vi "Enable-Disable MovCor UI.vi"(10 "MC Supported":bool) -> ()   [LabVIEW 2020]
uses:
  Global Variables/gl_UI Ctrl Refs.vi
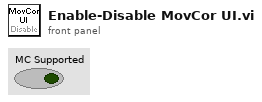
[diagram p1: front panel]
types:
  T1 = typedef "UI ctrl refs cluster.ctl" = cluster{"Top level VI path":path, "Top level VI ref":refnum<vi>, "User menu ref":refnum<k9>, "Sub Panel control":refnum<vi>, "Imaging Param Tab":refnum<vi>, "Occurrence-Start drivers":refnum<k4>, "Occurrence-Speed logging initialised":refnum<k4>, "Occurrence-XYZ stage initialised":refnum<k4>, "Exit button":refnum<vi>, "Status ind":refnum<vi>, "Set as origin":refnum<vi>, "Speed Logging":refnum<vi>, "Time Lapse":refnum<vi>, "Live Imaging":refnum<vi>, "AOL Z Stack":refnum<vi>, "Motor Z Stack":refnum<vi>, "Funct Acq button":refnum<vi>, "Hard Shutter":refnum<vi>, "Virtual Shutter":refnum<vi>, "Laser Power":refnum<vi>, "AOL Mode":refnum<vi>, "Frame Size":refnum<vi>, "Field of View":refnum<vi>, "Dwell Time":refnum<vi>, "Zoom":refnum<vi>, "AOL Z":refnum<vi>, "Objective":refnum<vi>, "Axis":refnum<vi>, "Paths & Names":refnum<vi>, "Experiment folder path (ind.)":refnum<vi>, "Last State (Ind.)":refnum<vi>, "Averages":refnum<vi>, "Angle (degrees)":refnum<vi>, "X centre":refnum<vi>, "Y centre":refnum<vi>, "Plane Mode":refnum<vi>, "# Planes":refnum<vi>, "Z Start":refnum<vi>, "Z Stop":refnum<vi>, "Z Step":refnum<vi>, "PMT 1":refnum<vi>, "PMT 2":refnum<vi>, "Stage XYZ Position":refnum<vi>, "Pockels@Z Start":refnum<vi>, "Pockels@Z Stop":refnum<vi>, "Obtain Z Start":refnum<vi>, "Obtain Z Stop":refnum<vi>, "Live stim.trig.period":refnum<vi>, "Live stim.trig.enable":refnum<vi>, "Movement Correction":refnum<vi>, "Load Reference Image":refnum<vi>, "XY Stage Move":refnum<vi>, "MovCor Cluster":refnum<vi>, "RefDAQParam":refnum<vi>, "Funct. Acq. Pockels Modulation":refnum<vi>, "Ref Laser Power":refnum<vi>, "Enable Video Recording":refnum<vi>, "Video Record-Live Imaging":refnum<vi>, "Video Record-Funct acq":refnum<vi>, "Reference Source":refnum<vi>, "AOL Z-stack Chirps Ready (ind)":refnum<vi>, "Target time between mov.cor. ref triggers (ms)":refnum<vi>, "Funct. Acq. Ref frame save":refnum<vi>, "Tracking button":refnum<vi>, "Show ref plots window":refnum<vi>, "Center freq ind (nm)":refnum<vi>, "Pickup mode (ind)":refnum<vi>, "Logging queue (ind)":refnum<vi>, "Back aperture power (ind.)":refnum<vi>, "Power after objective (ind.)":refnum<vi>, "Switch user":refnum<vi>, "Ls1 Conn. Status":refnum<vi>, "Ls1Tuning Status":refnum<vi>, "Ls1 Faults":refnum<vi>, "Ls1 Connection":refnum<vi>, "Ls1 Mode":refnum<vi>, "Ls1 POWER [mW]":refnum<vi>, "Ls1Shutter":refnum<vi>, "Ls1 Wavelength":refnum<vi>, "Ls1 Note":refnum<vi>, "Ls1 Confirm Wav":refnum<vi>, "Ls1 PreChrp Prism1":refnum<vi>, "Ls1 PreChrp Prism2":refnum<vi>, "Ls1 wav top Ind":refnum<vi>, "Ls1 power top Ind":refnum<vi>, "Ls1 Pump peak Hold":refnum<vi>, "Ls1 Status Ind":refnum<vi>, "Ls1 wav cancel":refnum<vi>, "Experiment Type":refnum<vi>, "Biology Information":refnum<vi>, "Camera recording status":refnum<vi>}
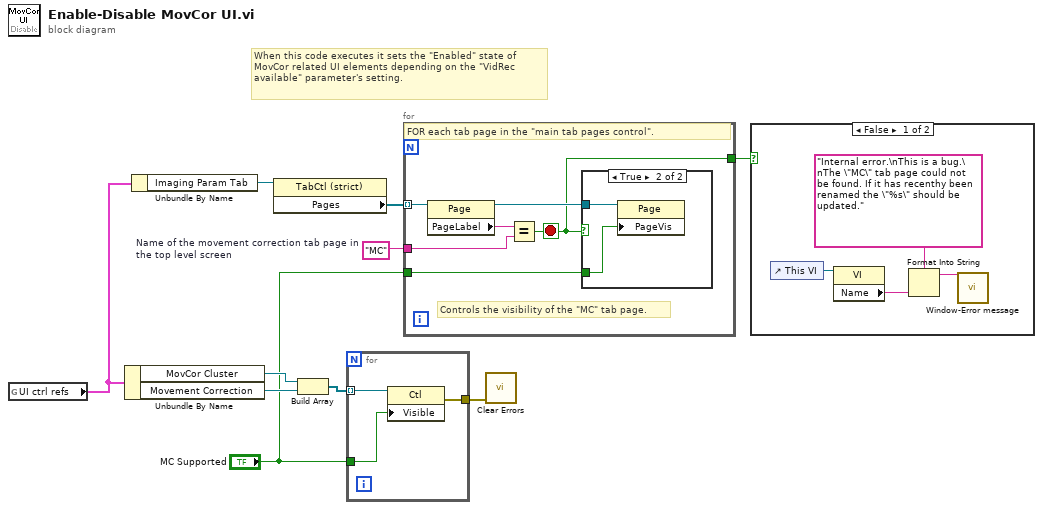
[diagram p0: block diagram]
diagram:
  w2 = "MC"  # Name of the movement correction tab page in the top level screen
  # "When this code executes it sets the \"Enabled\" state of MovCor related UI elements depending on the \"VidRec available\" parameter's setting."
  n1 = global read "gl_UI Ctrl Refs.vi" "UI ctrl refs"() -> (w6:T1)
  n2 = Unbundle By Name(w6) -> ("MovCor Cluster"=w10:refnum<vi>, "Movement Correction"=w9:refnum<vi>)
  n3 = Unbundle By Name(w6) -> ("Imaging Param Tab"=w5:refnum<vi>)
  n4 = property class="TabCtl (strict)"(reference=w5) -> ("Pages"=w4:refnum<vi>[])  [unwired: 1 in, 2 out]
  n5 = Build Array(w10, w9) -> (w8:refnum<vi>[])
  n6 = for {
    tunnel: w8 -> [w13] mode=indexing
    tunnel: "MC Supported" -> [w12]
    tunnel: [w11] -> w7
    n7 = property class="Ctl"(reference=w13, "Visible"=w12) -> (error out=w11:errorcluster)  [unwired: 1 in, 1 out]
  }
  n8 = for {
    tunnel: w4 -> [w19] mode=indexing
    tunnel: "MC Supported" -> [w16]
    tunnel: [w15] -> w3
    tunnel: w2 -> [w14]
    stop <- w15 stop-if-true
    # "Controls the visibility of the \"MC\" tab page."
    # "FOR each tab page in the \"main tab pages control\"."
    n9 = property class="Page"(reference=w19) -> (reference out=w17:refnum<vi>, "PageLabel"=w18:string)  [unwired: 1 in, 1 out]
    n10 = Equal?(x=w18, y=w14) -> (x = y?=w15:bool)
    n11 = case shown="True" w15 {
      tunnel: w17 -> [_ w21]
      tunnel: w16 -> [_ w20]
      frame False {
      }
      frame True {
        n12 = property class="Page"(reference=w21, "PageVis"=w20) -> ()  [unwired: 1 in, 2 out]
      }
    }
  }
  n13 = call <vilib>:"Clear Errors.vi"("error in (no error)"=w7) -> ()  [unwired: 5 in, 2 out]
  n14 = case shown="False" w3 {
    frame False {
      n15 = control-ref of="This VI"() -> (w25:refnum<vi>)
      n16 = property class="VI"(reference=w25) -> ("Name"=w23:string)  [unwired: 1 in, 2 out]
      n17 = Format Into String(format string="Internal error.\nThis is a bug.\nThe \"MC\" tab page could not be found. If it has recenthy been renamed the \"%s\" should be updated." ("Message"), w23) -> (resulting string=w22:string)  [unwired: 2 in, 1 out]
      n18 = call "Window-Error message.vi"("Message"=w22) -> ()  [unwired: 10 in, 1 out]
    }
    frame True {
    }
  }
